vi "End routeguide_RouteGuide_RecordRoute.vi"(8 "error in":errorcluster, 11 "Call ID in":T3) -> (0 "error out":errorcluster, 1 "errorDetails":T1, 2 "Response Data":T2)   [LabVIEW 2019, in "route_guide_client.lvlib"]
uses:
  route_guide_client.lvlib
  2435b599-b0f7-48e4-804e-62ee509d3e35.vi
  RPC Messages/routeguide_RouteSummary.ctl
  <vilib>/gRPC/LabVIEW gRPC Library/Shared/grpcId.ctl
  <vilib>/gRPC/LabVIEW gRPC Library/grpc-lvsupport-release.lvlib
  <vilib>/gRPC/LabVIEW gRPC Library/Shared/Any.ctl
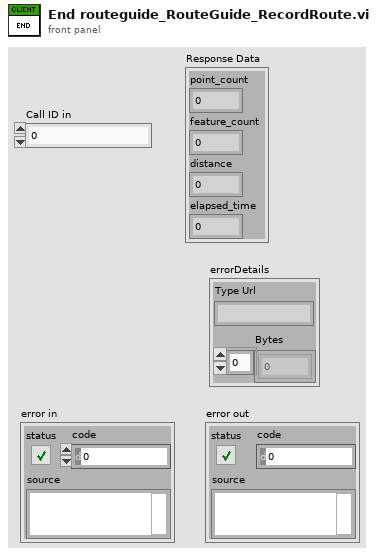
[diagram p1: front panel]
types:
  T1 = typedef "grpc-lvsupport-release.lvlib/Any.ctl" = cluster{"Type Url":string, "Bytes":u8[]}
  T2 = typedef "route_guide_client.lvlib/routeguide_RouteSummary.ctl" = cluster{"point_count":i32, "feature_count":i32, "distance":i32, "elapsed_time":i32}
  T3 = typedef "grpc-lvsupport-release.lvlib/grpcId.ctl" = u64
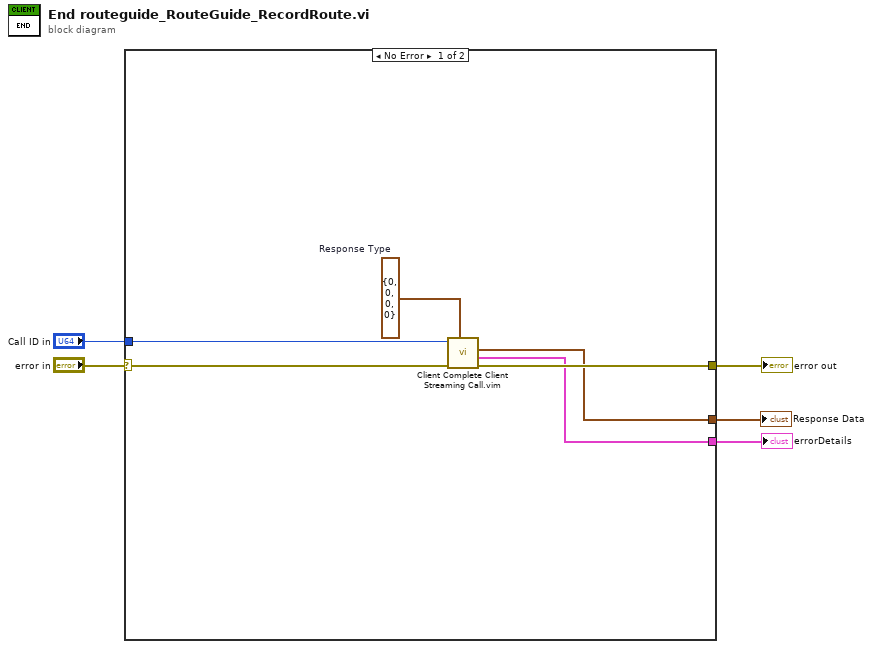
[diagram p0: block diagram]
diagram:
  n1 = case shown="No Error" "error in" {
    selector: "error in" -> [w11 w12]
    tunnel: [w10 w12] -> w4
    tunnel: "Call ID in" -> [w9 _]
    tunnel: [w8 _] -> w2
    tunnel: [w7 _] -> w1
    frame No Error {
      w6 = T2 {"point_count"=0, "feature_count"=0, "distance"=0, "elapsed_time"=0}  # Response Type
      n2 = call "Client Complete Client Streaming Call.vim"("Response Type"=w6, "error in"=w11, "Call ID in"=w9) -> ("error out"=w10:errorcluster, "errorDetails"=w7:T1, "Response Data"=w8:T2)  [unwired: 6 in]
    }
    frame Error {
    }
  }
  "error out" <- w4
  "Response Data" <- w2
  "errorDetails" <- w1
